vi "Write UnFiltered FIFO 2 RT with Sync Guard.vi"(9 "Sync Guard Data":fxp<+/-,38,12>[](array[numeric])=[888.2284999489784, 399.7682446986437, -617.0920498371124] format="%.9g", 10 "Raw Array Out":T1[](array[typedef])=[0.0, 0.0, 0.0, 0.0, 0.0, 0.0, 0.0, 0.0, 0.0, 0.0, 0.0, 0.0, 0.0, 0.0, 0.0, 0.0, 0.0, 0.0, 0.0, 0.0, 0.0, 0.0, 0.0, 0.0, 0.0, 0.0, 0.0, 0.0, 0.0, 0.0, 0.0, 0.0, 0.0, 0.0, 0.0, 0.0, 0.0, 0.0, 0.0, 0.0, 0.0, 0.0, 0.0, 0.0, 0.0, 0.0, 0.0, 0.0, 0.0, 0.0, 0.0, 0.0, 0.0, 0.0] format="%_6g") -> (3 "Timeout":bool)   [LabVIEW 2020]
doc: "Author: Scott Hannahs <sth@magnet.fsu.edu>\nCopyright 2018 Florida State University, All rights reserved."
uses:
  SCH Data Controls/SCH Data 2 RT.ctl
  <vilib>/rvi/interface/RandomDataEmulation/niFpgaRandomDataHandleErrors.vi
  <vilib>/rvi/DataTransferAndStorage/Container/XNode/niFpgaContainer.xnode
  <vilib>/rvi/interface/RandomDataEmulation/nirviRandomDataFpgaReadWriteTemplate.vi
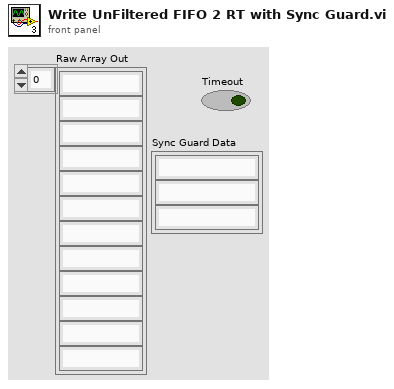
[diagram p1: front panel]
types:
  T1 = typedef "SCH Data 2 RT.ctl" = fxp<+/-,38,12>
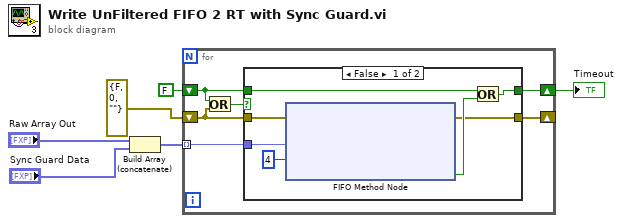
[diagram p0: block diagram]
diagram:
  n1 = Build Array (concatenate)("Raw Array Out", "Sync Guard Data") -> (w4:T1[])
  n2 = for {
    tunnel: w4 -> [w12] mode=indexing
    shift-right: [w11] -> w5
    shift-left: FALSE -> [w9]
    shift-right: [w10] -> _
    shift-left: errorcluster {"Status?"=FALSE, "Code"=0, "Source"=""} ("error out") -> [w8]
    n3 = Or(x=w9, y=w8) -> (x .or. y?=w7:bool)
    n4 = case shown="False" w7 {
      tunnel: w12 -> [w19 _]
      tunnel: [w17 w20] -> w11
      tunnel: w9 -> [w16 w20]
      tunnel: w8 -> [w14 w21]
      tunnel: [w13 w21] -> w10
      frame False {
        n5 = xnode ("FIFO Method Node")("Element"=w19, "Timeout"=4, "error in (no error)"=w14) -> ("Timed Out?"=w18:bool, "error out"=w13:errorcluster)  [unwired: 1 in, 1 out]
        n6 = Or(x=w16, y=w18) -> (x .or. y?=w17:bool)
      }
      frame True {
      }
    }
  }
  "Timeout" <- w5
